vi "Write Serial Data.vi"(8 "error in":errorcluster, 10 "CRD Data In":refnum<class "CRDS Data.lvclass">=refnum, 11 "File Obs in":refnum<class "CRD File Obs.lvclass">) -> (0 "error out":errorcluster, 2 "CRD Data Out":refnum<class "CRDS Data.lvclass">, 3 "File Obs Out":refnum<class "CRD File Obs.lvclass">)   [LabVIEW 2014, in "CRD File Obs.lvclass"]
uses:
  CRD File Obs.lvclass
  Devices/Alicat/Data/MC/AlicatMCData.lvclass
  Data/Main/CRDS Data.lvclass
  Data/Main/crd_data_enum.ctl
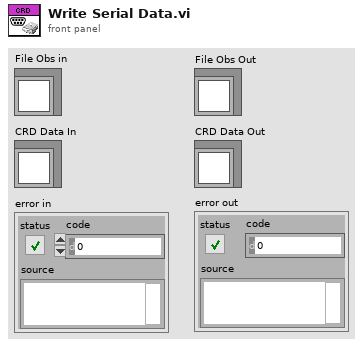
[diagram p1: front panel]
types:
  T1 = enum16{"big-endian, network order", "native, host order", "little-endian"}
  T2 = cluster{"P":sgl, "T":sgl, "Q":sgl, "Q0":sgl, "Qsp":sgl}
  T3 = typedef "crd_data_enum.ctl" = enum8{"Time", "RHw", "TRH", "P", "Tmean", "RHsense", "TQ", "PQ", "Q", "Q0", "Qcal", "Qset", "extDilFac", "taucorr", "tau0corr", "stdevtau", "ext", "extCorr", "etau", "tau", "tau0", "Purge_Data", "NoData", "reserved", "Ttec", "Ang Exp", "Gamma", "filter", "fOverride", "notes", "max amp", "Tthermistor", "RhdilFac", "Psense", "TRHsense_bank", "RHsense_bank", "MFC_Data", "Thum", "ThumSP", "O3 Flow", "Pinlet Flow", "CLAP Flow", "O3 Add Valve", "O2 Valve", "O3 Cal"}
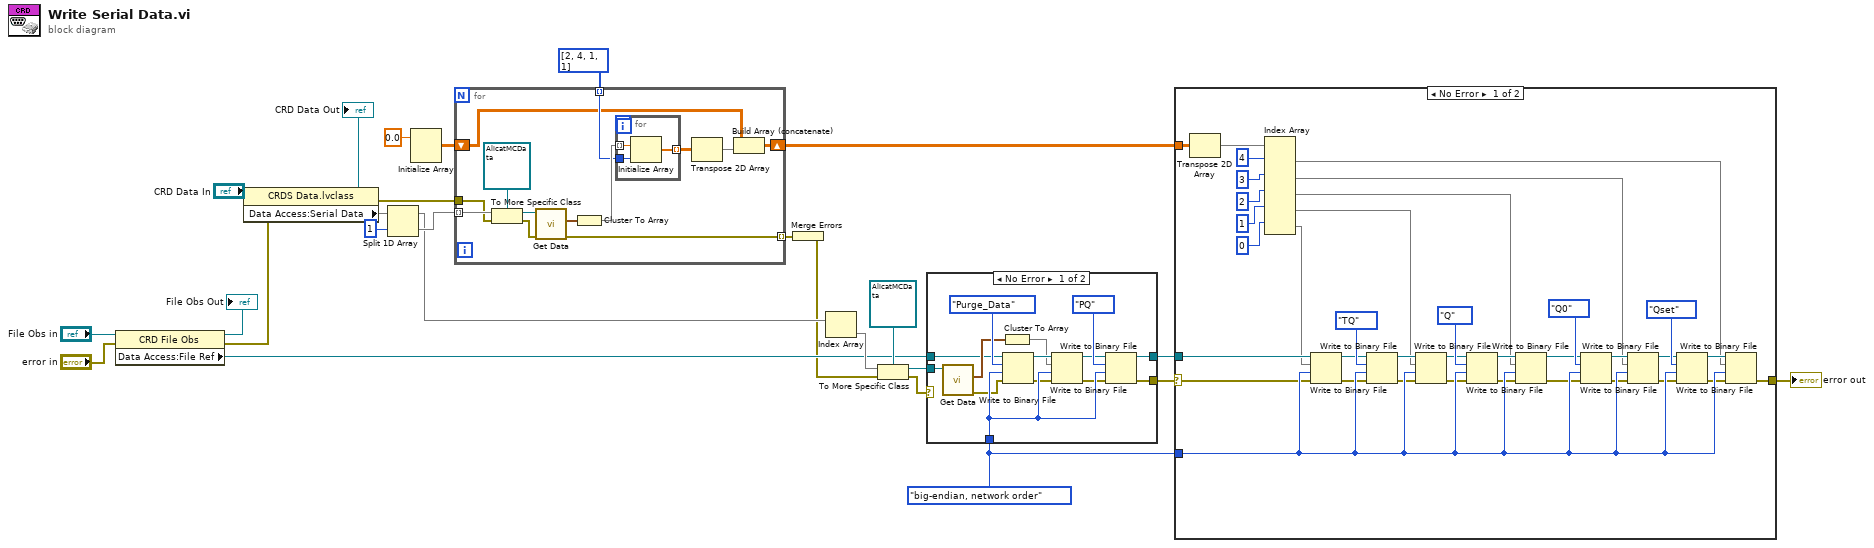
[diagram p0: block diagram]
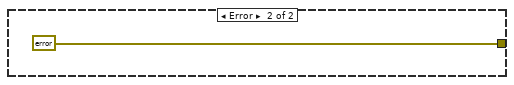
[diagram p2: hidden frame]
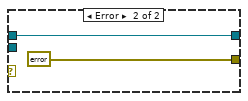
[diagram p3: hidden frame]
diagram:
  w20 = T1."big-endian, network order" ("byte order (0:big-endian, network order)")
  n1 = property class="CRD File Obs"(reference="File Obs in", error in="error in") -> (reference out=→"File Obs Out":refnum<class "CRD File Obs.lvclass">, error out=w2:errorcluster, "Data Access:File Ref"=w12:refnum<file>)
  n2 = property class="CRDS Data.lvclass"(reference="CRD Data In", error in=w2) -> (reference out=→"CRD Data Out":refnum<class "CRDS Data.lvclass">, error out=w8:errorcluster, "Data Access:Serial Data"=w11)
  n3 = Split 1D Array(array=w11, index=1) -> (first subarray=w21:void[], second subarray=w24:void[])
  n4 = Initialize Array(sgl 0.0 ("element")) -> (w19:sgl[][])  [unwired: 2 in]
  n5 = for {
    tunnel: w24 -> [w36] mode=indexing
    tunnel: i32[] [2, 4, 1, 1] -> [w33] mode=indexing
    shift-right: [w29] -> w5
    shift-left: w19 -> [w30]
    tunnel: [w28] -> w26 mode=indexing
    tunnel: w8 -> [w27]
    n6 = To More Specific Class(target class=refnum<class "AlicatMCData.lvclass"> refnum ("Alicat.lvlib:AlicatMCData.lvclass"), reference=w36, error in=w27) -> (specific class reference=w38:refnum<class "AlicatMCData.lvclass">, error out=w37:errorcluster)
    n7 = call "Get Data.vi"("error in"=w37, "AlicatMData in"=w38) -> ("error out"=w28:errorcluster, "SystemData"=w35:T2)  [unwired: 7 in, 1 out]
    n8 = Cluster To Array(cluster=w35) -> (array=w34:sgl[])
    n9 = for {
      tunnel: w34 -> [w42] mode=indexing
      tunnel: w33 -> [w41]
      tunnel: [w40] -> w32 mode=indexing
      n10 = Initialize Array(w42, w41) -> (w40:sgl[])
    }
    n11 = Transpose 2D Array(2D array=w32) -> (transposed array=w31:sgl[][])
    n12 = Build Array (concatenate)(w30, w31) -> (w29:sgl[][])
  }
  n13 = Merge Errors(w26) -> (w7:errorcluster)
  n14 = Index Array(array=w21) -> (element=w23)  [unwired: 1 in]
  n15 = To More Specific Class(target class=refnum<class "AlicatMCData.lvclass"> refnum ("Alicat.lvlib:AlicatMCData.lvclass"), reference=w23, error in=w7) -> (specific class reference=w15:refnum<class "AlicatMCData.lvclass">, error out=w25:errorcluster)
  n16 = case shown="No Error" w25 {
    tunnel: w15 -> [w56 _]
    tunnel: w20 -> [w55 _]
    tunnel: [w52 errorcluster {"status"=FALSE, "code"=0, "source"=""} ("error out")] -> w4
    tunnel: [w51 w57] -> w13
    tunnel: w12 -> [w43 w57]
    frame No Error {
      n17 = call "Get Data.vi"("AlicatMData in"=w56) -> ("error out"=w48:errorcluster, "SystemData"=w47:T2)  [unwired: 8 in, 1 out]
      n18 = Cluster To Array(cluster=w47) -> (array=w46:sgl[])
      n19 = Write to Binary File(file (use dialog)=w43, data=crd_data_enum."Purge_Data" ("CRD_Data_Enum"), error in=w48, 9:w55) -> (refnum out=w54:refnum<file>, error out=w49:errorcluster)  [unwired: 2 in, 1 out]
      n20 = Write to Binary File(file (use dialog)=w54, data=w46, error in=w49, 9:w55) -> (refnum out=w45:refnum<file>, error out=w44:errorcluster)  [unwired: 2 in, 1 out]
      n21 = Write to Binary File(file (use dialog)=w45, data=crd_data_enum."PQ" ("CRD_Data_Enum"), error in=w44, 9:w55) -> (refnum out=w51:refnum<file>, error out=w52:errorcluster)  [unwired: 2 in, 1 out]
    }
    frame Error {
    }
  }
  n22 = case shown="No Error" w4 {
    selector: w4 -> [w59 _]
    tunnel: w20 -> [w94 _]
    tunnel: [w93 errorcluster {"status"=FALSE, "code"=0, "source"=""} ("error out")] -> w6
    tunnel: w13 -> [w92 _]
    tunnel: w5 -> [w61 _]
    frame No Error {
      n23 = Transpose 2D Array(2D array=w61) -> (transposed array=w60:sgl[][])
      n24 = Index Array(array=w60, index (row) #1=4 ("index (row)"), index (row) #2=3 ("index (row)"), index (row) #3=2 ("index (row)"), index (row) #4=1 ("index (row)"), index (row) #5=0 ("index (row)")) -> (element #1=w66:sgl[], element #2=w65:sgl[], element #3=w64:sgl[], element #4=w63:sgl[], element #5=w62:sgl[])  [unwired: 5 in]
      n25 = Write to Binary File(file (use dialog)=w92, data=w62, error in=w59, 9:w94) -> (refnum out=w88:refnum<file>, error out=w87:errorcluster)  [unwired: 2 in, 1 out]
      n26 = Write to Binary File(file (use dialog)=w88, data=crd_data_enum."TQ" ("CRD_Data_Enum"), error in=w87, 9:w94) -> (refnum out=w91:refnum<file>, error out=w90:errorcluster)  [unwired: 2 in, 1 out]
      n27 = Write to Binary File(file (use dialog)=w91, data=w63, error in=w90, 9:w94) -> (refnum out=w83:refnum<file>, error out=w82:errorcluster)  [unwired: 2 in, 1 out]
      n28 = Write to Binary File(file (use dialog)=w83, data=crd_data_enum."Q" ("CRD_Data_Enum"), error in=w82, 9:w94) -> (refnum out=w85:refnum<file>, error out=w86:errorcluster)  [unwired: 2 in, 1 out]
      n29 = Write to Binary File(file (use dialog)=w85, data=w64, error in=w86, 9:w94) -> (refnum out=w78:refnum<file>, error out=w77:errorcluster)  [unwired: 2 in, 1 out]
      n30 = Write to Binary File(file (use dialog)=w78, data=crd_data_enum."Q0" ("CRD_Data_Enum"), error in=w77, 9:w94) -> (refnum out=w81:refnum<file>, error out=w80:errorcluster)  [unwired: 2 in, 1 out]
      n31 = Write to Binary File(file (use dialog)=w81, data=w65, error in=w80, 9:w94) -> (refnum out=w73:refnum<file>, error out=w72:errorcluster)  [unwired: 2 in, 1 out]
      n32 = Write to Binary File(file (use dialog)=w73, data=crd_data_enum."Qset" ("CRD_Data_Enum"), error in=w72, 9:w94) -> (refnum out=w75:refnum<file>, error out=w76:errorcluster)  [unwired: 2 in, 1 out]
      n33 = Write to Binary File(file (use dialog)=w75, data=w66, error in=w76, 9:w94) -> (error out=w93:errorcluster)  [unwired: 2 in, 2 out]
    }
    frame Error {
    }
  }
  "error out" <- w6
